vi "Get Fix Velocity.vi"(8 "error in (no error)":errorcluster, 11 "nmea in":refnum<class "nmea.lvclass">) -> (0 "error out":errorcluster, 2 "Fix Velocity":T1 {"Fix"."Longitude" format="%_16f"; "Fix"."Latitude" format="%_16f"}, 3 "nmea out":refnum<class "nmea.lvclass">)   [LabVIEW 2020, in "nmea.lvlib" / "nmea.lvclass"]
uses:
  nmea.lvclass
  Fix Velocity.ctl
  Fix.ctl
  Velocity.ctl
  nmea.lvclass/nmea.ctl
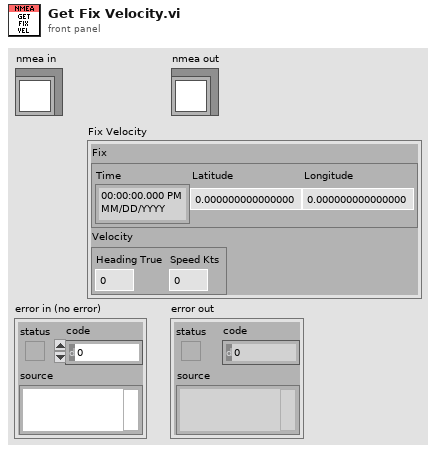
[diagram p1: front panel]
types:
  T1 = typedef "nmea.lvlib/nmea.lvclass/Fix Velocity.ctl" = cluster{"Fix":T2, "Velocity":T3}
  T2 = typedef "nmea.lvlib/nmea.lvclass/Fix.ctl" = cluster{"Time":timestamp, "Latitude":dbl, "Longitude":dbl}
  T3 = typedef "nmea.lvlib/nmea.lvclass/Velocity.ctl" = cluster{"Heading True":dbl, "Speed Kts":dbl}
  T4 = typedef "nmea.lvlib/nmea.lvclass/Ref Data.ctl" = cluster{"Latitude":dbl, "Longitude":dbl, "Time":T5, "Status":string, "Speed":dbl, "Course":dbl, "Mag Var":dbl, "Var Dir":string, "Mode":string, "Satellites":T6[], "Next Satellites":T6[], "Active PRNs":i32[], "Fix Type":T7, "DOP":T8, "Fix Mode":T9, "Altitude":dbl, "Geoid":dbl}
  T5 = typedef "LVDateTimeRec.ctl" = cluster{"fractional second":dbl, "second":i32, "minute":i32, "hour":i32, "day of month":i32, "month":i32, "year":i32, "day of week":i32, "day of year":i32, "DST":i32}
  T6 = typedef "nmea.lvlib/nmea.lvclass/Satellite.ctl" = cluster{"PRN":u8, "Channel":u8, "Elevation":u8, "Azimuth":u16, "SNR":u8, "Active":bool}
  T7 = typedef "nmea.lvlib/nmea.lvclass/Fix Type.ctl" = enum16{"N/A", "None", "2D", "3D"}
  T8 = typedef "nmea.lvlib/nmea.lvclass/DOP.ctl" = cluster{"P":dbl, "H":dbl, "V":dbl}
  T9 = typedef "nmea.lvlib/nmea.lvclass/Fix Mode.ctl" = enum16{"Manual", "Auto 2/3D"}
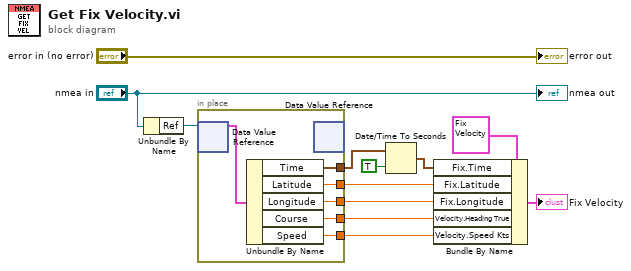
[diagram p0: block diagram]
diagram:
  n1 = Unbundle By Name("nmea in") -> ("Ref"=w11:refnum<data-value>)
  n2 = in-place {
    in-place-border: [w17] -> w9
    in-place-border: [w16] -> w6
    in-place-border: [w15] -> w5
    in-place-border: [w14] -> w4
    in-place-border: [w13] -> w3
    n3 = in-place-dvr #1(w11) -> (w18:T4)  [unwired: 1 out]
    n4 = Unbundle By Name(w18) -> ("Time"=w17:T5, "Latitude"=w16:dbl, "Longitude"=w15:dbl, "Course"=w14:dbl, "Speed"=w13:dbl)
    n5 = in-place-dvr #1() -> ()  [unwired: 1 in, 2 out]
  }
  n6 = Date/Time To Seconds(1:TRUE ("is UTC (F)"), 2:w9) -> (0:w2:timestamp)
  n7 = Bundle By Name(cluster=T1 {"Fix"={"Time"=timestamp(0 s since 1904-01-01), "Latitude"=0.0, "Longitude"=0.0}, "Velocity"={"Heading True"=0.0, "Speed Kts"=0.0}} ("Fix Velocity"), "Fix.Time"=w2, "Fix.Latitude"=w6, "Fix.Longitude"=w5, "Velocity.Heading True"=w4, "Velocity.Speed Kts"=w3) -> (→"Fix Velocity":T1)
  "error out" <- "error in (no error)"
  "nmea out" <- "nmea in"
